vi "ex13-2.vi"   [LabVIEW 2009]
uses:
  <vilib>/NXT/Block Support/NXT_InputPort.ctl
  <vilib>/NXT/Subs/MotorOutput.ctl
  C:/Program Files/National Instruments/mindsensors/mindsensors.com LVEE Toolkit/Dual/NXTCam-DM.vi
  <vilib>/NXT/Dual Mode Library/Motors/MotorReverse.vi
types:
  T1 = cluster{"Tracking Mode":u8, "Object Number to Track":u8}
  T2 = typedef "NXT_InputPort.ctl" = u8
  T3 = typedef "LVHSConnector.ctl" = cluster{"error":errorcluster, "address":string, "NXT #":i32, "Show Error":bool, "Connection":u16}
  T4 = typedef "MotorOutput.ctl" = u8
  T5 = cluster{"Total Tracked Objects":u8, "Color":u8, "X Upper Left":u8, "Y Upper Left":u8, "X Lower Right":u8, "Y Lower Right":u8, "Status (boolean)":bool}
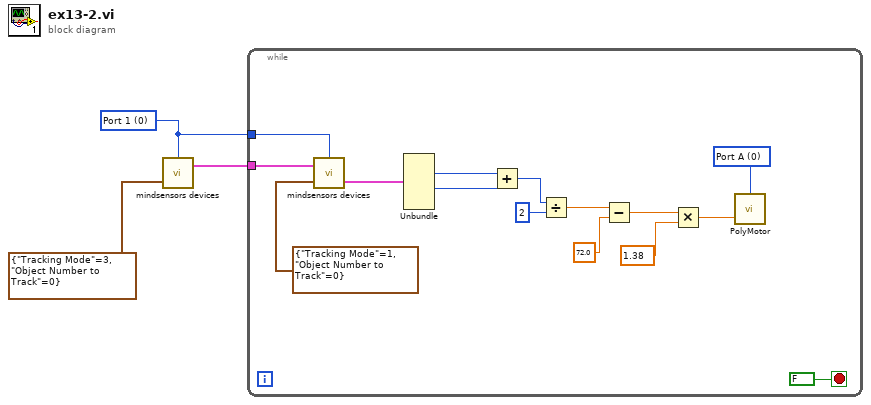
[diagram p0: block diagram]
diagram:
  w2 = T2 0 items=["Port 1", "Port 2", "Port 3", "Port 4"] ("Input Port")
  n1 = call-poly "mindsensors devices.vi"("Input of NXTCam"=T1 {"Tracking Mode"=3, "Object Number to Track"=0}, "Input Port"=w2) -> ("NXT dup"=w3:T3)  [unwired: 1 in, 1 out]
  n2 = while {
    tunnel: w3 -> [w17]
    tunnel: w2 -> [w16]
    stop <- FALSE stop-if-true
    w5 = T4 0 items=["Port A", "Port B", "Port C", "All Ports"] ("Output Port (All Ports)")
    n3 = call-poly "mindsensors devices.vi"("Input of NXTCam"=T1 {"Tracking Mode"=1, "Object Number to Track"=0}, "NXT"=w17, "Input Port"=w16) -> ("Output of NXTCam"=w14:T5)  [unwired: 1 out]
    n4 = Unbundle(w14) -> ("X Upper Left"=w13:u8, "X Lower Right"=w12:u8)  [unwired: 5 out]
    n5 = Add(x=w13, y=w12) -> (x+y=w11:u8)
    n6 = Divide(x=w11, y=u8 2) -> (x/y=w9:dbl)
    n7 = Subtract(x=w9, y=72.0) -> (x-y=w7:dbl)
    n8 = Multiply(x=w7, y=1.38) -> (x*y=w4:dbl)
    n9 = call-poly <vilib>:"PolyMotor.vi"("Power (75)"=w4, "Output Port (All Ports)"=w5) -> ()  [unwired: 2 in, 1 out]
  }
